vi "Configure Safety Settings.vi"(0 "VISA resource name":refnum<visa-resource-name>, 5 "Motor ID (0)":u8, 7 "Alarm Settings":cluster{"LED Alarm":T1, "Shutdown Alarm":T1}={"LED Alarm"={"Input Voltage"=TRUE, "Angle Limit"=FALSE, "Overheating "=TRUE, "Range"=FALSE, "Checksum"=FALSE, "Overload"=FALSE, "Instruction"=FALSE}, "Shutdown Alarm"={"Input Voltage"=TRUE, "Angle Limit"=FALSE, "Overheating "=TRUE, "Range"=FALSE, "Checksum"=FALSE, "Overload"=FALSE, "Instruction"=FALSE}}, 9 "Safety Limits":T2={"Temperature Limit (C)"=80, "Low Voltage Limit (V)"=5.0, "High Voltage Limit (V)"=25.0, "Maximum Torque%"=100.0}, 11 "error in (no error)":errorcluster) -> (4 "VISA resource name out":refnum<visa-resource-name>, 15 "error out":errorcluster)   [LabVIEW 2016, in "Dynamixel Motor.lvlib"]
doc: "Sets limits for the temperature, voltage, and torque for the motor as well as the action to take for status errors for: temperature, overload, angle limit, checksum, etc."
uses:
  Dynamixel Motor.lvlib
  Motor Operation/Low Level/Alarm Setting.ctl
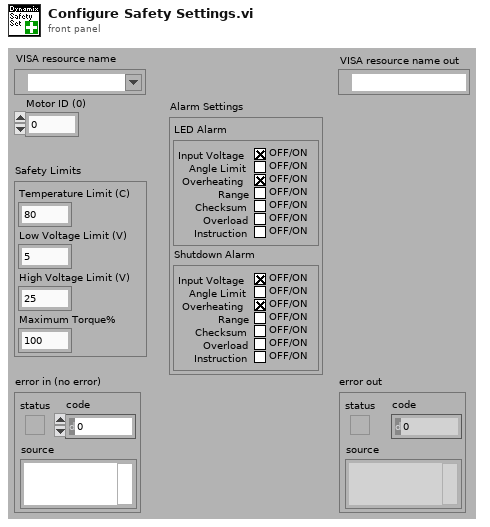
[diagram p1: front panel]
types:
  T1 = typedef "Dynamixel Motor.lvlib/Alarm Setting.ctl" = cluster{"Input Voltage":bool, "Angle Limit":bool, "Overheating ":bool, "Range":bool, "Checksum":bool, "Overload":bool, "Instruction":bool}
  T2 = cluster{"Temperature Limit (C)":u8, "Low Voltage Limit (V)":dbl, "High Voltage Limit (V)":dbl, "Maximum Torque%":dbl}
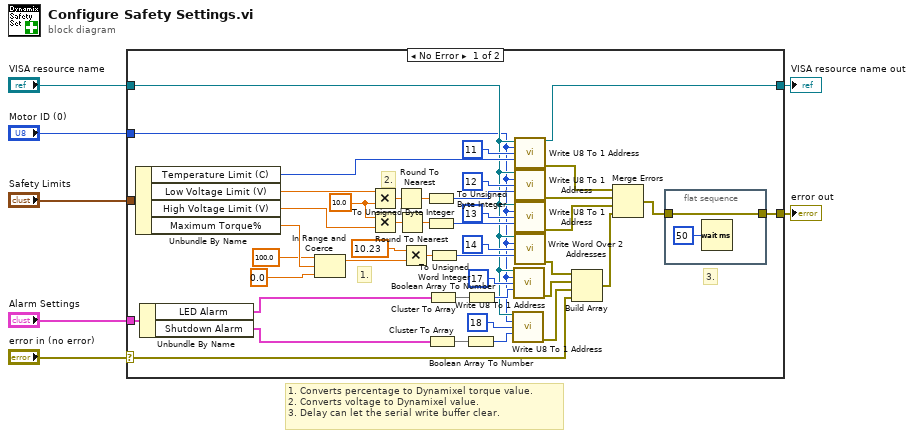
[diagram p0: block diagram]
diagram:
  # "1. Converts percentage to Dynamixel torque value.\n2. Converts voltage to Dynamixel value.\n3. Delay can let the serial write buffer clear."
  n1 = case shown="No Error" "error in (no error)" {
    selector: "error in (no error)" -> [w19 w55]
    tunnel: "VISA resource name" -> [w15 w54]
    tunnel: "Motor ID (0)" -> [w14 _]
    tunnel: [w13 w54] -> w1
    tunnel: "Safety Limits" -> [w44 _]
    tunnel: [w11 w55] -> w3
    tunnel: "Alarm Settings" -> [w23 _]
    frame No Error {
      w39 = 10.0 ("y")
      # "3."
      # "2."
      # "1."
      n2 = Unbundle By Name(w44) -> ("Temperature Limit (C)"=w43:u8, "Low Voltage Limit (V)"=w41:dbl, "High Voltage Limit (V)"=w40:dbl, "Maximum Torque%"=w33:dbl)
      n3 = Unbundle By Name(w23) -> ("LED Alarm"=w17:T1, "Shutdown Alarm"=w16:T1)
      n4 = In Range and Coerce(upper limit=100.0, x=w33, lower limit=0.0) -> (coerced(x)=w10:dbl)  [unwired: 1 out]
      n5 = Multiply(x=w41, y=w39) -> (x*y=w38:dbl)
      n6 = Multiply(x=w39, y=w40) -> (x*y=w42:dbl)
      n7 = Round To Nearest(number=w38) -> (nearest integer value=w36:dbl)
      n8 = Round To Nearest(number=w42) -> (nearest integer value=w37:dbl)
      n9 = Multiply(x=10.23, y=w10) -> (x*y=w47:dbl)
      n10 = To Unsigned Byte Integer(number=w36) -> (unsigned 8bit integer=w35:u8)
      n11 = To Unsigned Byte Integer(number=w37) -> (unsigned 8bit integer=w34:u8)
      n12 = Cluster To Array(cluster=w16) -> (array=w21:bool[])
      n13 = Cluster To Array(cluster=w17) -> (array=w31:bool[])
      n14 = To Unsigned Word Integer(number=w47) -> (unsigned 16bit integer=w45:u16)
      n15 = Boolean Array To Number(Boolean array=w21) -> (number=w22:u32)
      n16 = Boolean Array To Number(Boolean array=w31) -> (number=w30:u32)
      n17 = call "Write U8 To 1 Address.vi"("VISA resource name"=w15, "Motor ID (0)"=w14, "Address number (0)"=u8 18, "Parameter (0)"=w22) -> ("error out"=w18:errorcluster)  [unwired: 10 in, 1 out]
      n18 = call "Write U8 To 1 Address.vi"("VISA resource name"=w15, "Motor ID (0)"=w14, "Address number (0)"=u8 17, "Parameter (0)"=w30) -> ("error out"=w25:errorcluster)  [unwired: 10 in, 1 out]
      n19 = call "Write U8 To 1 Address.vi"("VISA resource name"=w15, "Motor ID (0)"=w14, "Address number (0)"=u8 11, "Parameter (0)"=w43) -> ("VISA resource name out"=w13:refnum<visa-resource-name>, "error out"=w29:errorcluster)  [unwired: 10 in]
      n20 = call "Write U8 To 1 Address.vi"("VISA resource name"=w15, "Motor ID (0)"=w14, "Address number (0)"=u8 12, "Parameter (0)"=w35) -> ("error out"=w28:errorcluster)  [unwired: 10 in, 1 out]
      n21 = call "Write U8 To 1 Address.vi"("VISA resource name"=w15, "Motor ID (0)"=w14, "Address number (0)"=u8 13, "Parameter (0)"=w34) -> ("error out"=w27:errorcluster)  [unwired: 10 in, 1 out]
      n22 = call "Write Word Over 2 Addresses.vi"("VISA resource name"=w15, "Motor ID (0)"=w14, "Address number (0)"=u8 14, "Parameter (0)"=w45) -> ("error out"=w26:errorcluster)  [unwired: 10 in, 1 out]
      n23 = Build Array(w26, w25, w18, w19) -> (w24:errorcluster[])
      n24 = Merge Errors(w29, w28, w27, w24) -> (w12:errorcluster)
      n25 = flat-sequence {
        tunnel: w12 -> [w52]
        tunnel: [w52] -> w11
        frame #0 {
          n26 = Wait (ms)(milliseconds to wait=u32 50) -> ()  [unwired: 1 out]
        }
      }
    }
    frame Error {
    }
  }
  "VISA resource name out" <- w1
  "error out" <- w3
